vi "SW_NumberToBoolArry.vi"(0 "L STR":string, 1 "H STR":string) -> (20 "H1":bool[](array[boolean]), 21 "H2":bool[](array[boolean]), 22 "H3":bool[](array[boolean]), 23 "H4":bool[](array[boolean]), 24 "L1":bool[](array[boolean]), 25 "L2":bool[](array[boolean]), 26 "L3":bool[](array[boolean]), 27 "L4":bool[](array[boolean]))   [LabVIEW 2018]
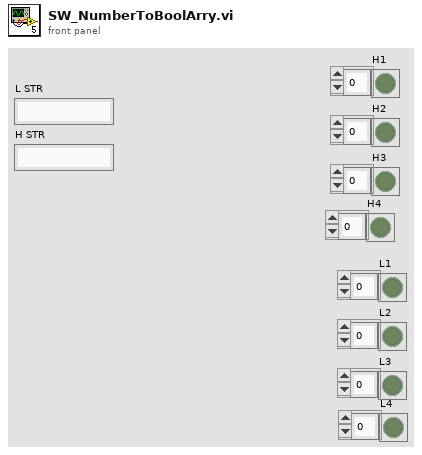
[diagram p1: front panel]
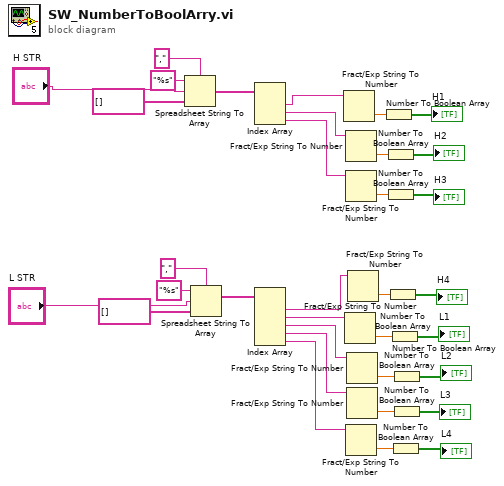
[diagram p0: block diagram]
diagram:
  n1 = Spreadsheet String To Array(delimiter (Tab)="," ("分隔符(Tab)"), format string="%s" ("格式字符串"), spreadsheet string="H STR", array type (2D Dbl)=string[] []) -> (array=w18:string[])
  n2 = Spreadsheet String To Array(delimiter (Tab)="," ("分隔符(Tab)"), format string="%s" ("格式字符串"), spreadsheet string="L STR", array type (2D Dbl)=string[] []) -> (array=w26:string[])
  n3 = Index Array(array=w18) -> (element #1=w23:string, element #2=w24:string, element #3=w25:string)  [unwired: 3 in]
  n4 = Index Array(array=w26) -> (element #1=w1:string, element #2=w27:string, element #3=w32:string, element #4=w33:string, element #5=w34:string)  [unwired: 5 in]
  n5 = Fract/Exp String To Number(string=w23) -> (number=w20:dbl)  [unwired: 3 in, 1 out]
  n6 = Fract/Exp String To Number(string=w27) -> (number=w29:dbl)  [unwired: 3 in, 1 out]
  n7 = Fract/Exp String To Number(string=w24) -> (number=w19:dbl)  [unwired: 3 in, 1 out]
  n8 = Fract/Exp String To Number(string=w25) -> (number=w21:dbl)  [unwired: 3 in, 1 out]
  n9 = Fract/Exp String To Number(string=w34) -> (number=w31:dbl)  [unwired: 3 in, 1 out]
  n10 = Fract/Exp String To Number(string=w32) -> (number=w28:dbl)  [unwired: 3 in, 1 out]
  n11 = Fract/Exp String To Number(string=w33) -> (number=w30:dbl)  [unwired: 3 in, 1 out]
  n12 = Fract/Exp String To Number(string=w1) -> (number=w22:dbl)  [unwired: 3 in, 1 out]
  n13 = Number To Boolean Array(number=w20) -> (Boolean array=→"H1":bool[])
  n14 = Number To Boolean Array(number=w19) -> (Boolean array=→"H2":bool[])
  n15 = Number To Boolean Array(number=w21) -> (Boolean array=→"H3":bool[])
  n16 = Number To Boolean Array(number=w22) -> (Boolean array=→"H4":bool[])
  n17 = Number To Boolean Array(number=w29) -> (Boolean array=→"L1":bool[])
  n18 = Number To Boolean Array(number=w31) -> (Boolean array=→"L4":bool[])
  n19 = Number To Boolean Array(number=w28) -> (Boolean array=→"L2":bool[])
  n20 = Number To Boolean Array(number=w30) -> (Boolean array=→"L3":bool[])
